vi "FrameToTag(array)__slk_mt.vi"(8 "error in (no error)":errorcluster, 10 "frames":string[](array[string]), 11 "numeric adapter in":refnum<class "NumericAdapter__slk_mt.lvclass">) -> (0 "error out":errorcluster, 2 "tags":string[](array[string]), 3 "numeric adapter out":refnum<class "NumericAdapter__slk_mt.lvclass">)   [LabVIEW 2012, in "Lazyboots Menu Tool.lvlib" / "NumericAdapter__slk_mt.lvclass"]
doc: "Converts case frame names to tree control tags."
uses:
  NumericAdapter__slk_mt.lvclass
panel:
  # "FrameToTag(array)__slk_mt.vi\nConverts case frame names to tree control tags.\n\nNOTICE -- YOU MUST LEAVE THIS NOTICE IN PLACE.\n\nCopyright (c) 2011, LIANG LIU Shawn.Liu.cn@gmail.com\nAll rights reserved.\n\nRedistribution and use in source and binary forms, with or without modification, are permitted provided that the following conditions are met:\n-Redistributions of source code must retain the above copyright notice, this list of conditions and the following disclaimer.\n-Redistributions in binary form must reproduce the above copyright notice, this list of conditions and the following disclaimer in the documentation and/or other materials provided with the distribution.\n-Neither the name of the eLp nor the names of its contributors may be used to endorse or promote products derived from this software without specific prior written permission.\n\nTHIS SOFTWARE IS PROVIDED BY THE COPYRIGHT HOLDERS AND CONTRIBUTORS \"AS IS\" AND ANY EXPRESS OR IMPLIED WARRANTIES, INCLUDING, BUT NOT LIMITED TO, THE IMPLIED WARRANTIES OF MERCHANTABILITY AND FITNESS FOR A PARTICULAR PURPOSE ARE DISCLAIMED. IN NO EVENT SHALL THE COPYRIGHT HOLDER OR CONTRIBUTORS BE LIABLE FOR ANY DIRECT, INDIRECT, INCIDENTAL, SPECIAL, EXEMPLARY, OR CONSEQUENTIAL DAMAGES (INCLUDING, BUT NOT LIMITED TO, PROCUREMENT OF SUBSTITUTE GOODS OR SERVICES; LOSS OF USE, DATA, OR PROFITS; OR BUSINESS INTERRUPTION) HOWEVER CAUSED AND ON ANY THEORY OF LIABILITY, WHETHER IN CONTRACT, STRICT LIABILITY, OR TORT (INCLUDING NEGLIGENCE OR OTHERWISE) ARISING IN ANY WAY OUT OF THE USE OF THIS SOFTWARE, EVEN IF ADVISED OF THE POSSIBILITY OF SUCH DAMAGE."
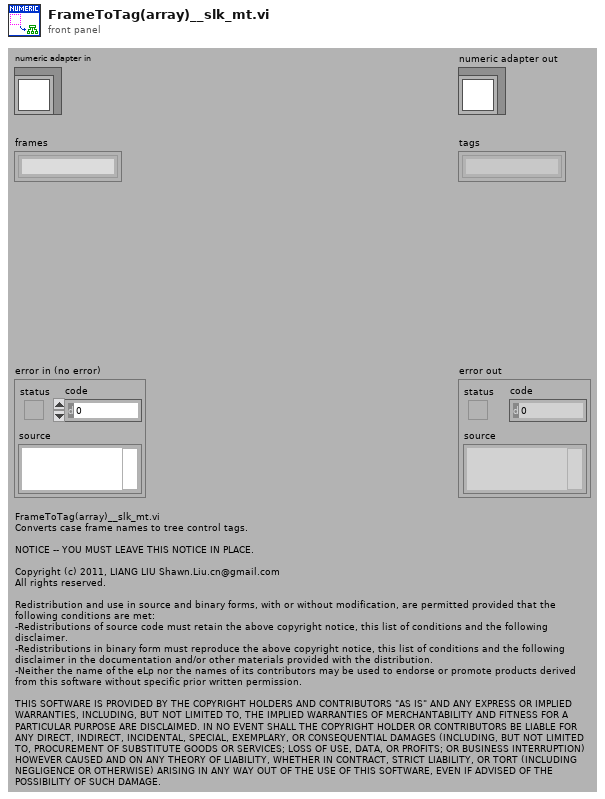
[diagram p1: front panel]
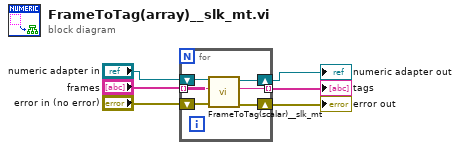
[diagram p0: block diagram]
diagram:
  n1 = for {
    shift-right: [w11] -> w6
    shift-left: "numeric adapter in" -> [w12]
    shift-right: [w9] -> w5
    shift-left: "error in (no error)" -> [w10]
    tunnel: "frames" -> [w8] mode=indexing
    tunnel: [w7] -> w2 mode=indexing
    n2 = call-dynamic "FrameToTag(scalar)__slk_mt.vi"("error in (no error)"=w10, "frame"=w8, "numeric adapter in"=w12) -> ("error out"=w9:errorcluster, "tag"=w7:string, "numeric adapter out"=w11:refnum<class "NumericAdapter__slk_mt.lvclass">)  [unwired: 6 in]
  }
  "error out" <- w5
  "numeric adapter out" <- w6
  "tags" <- w2
